vi "Synchronous Trigger (5772).vi"() -> (1 "Trigger":bool[](array[boolean]), 2 "Trigger":u8, 3 "Trig":bool)   [LabVIEW 2012]
uses:
  <vilib>/rvi/eio/common/nirviEmuTemplateMethod_errors.vi
  <vilib>/eio/EIONode/EIONode.xnode
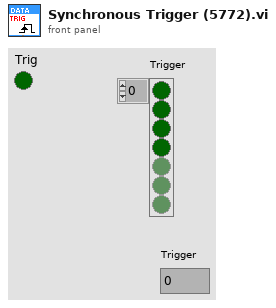
[diagram p1: front panel]
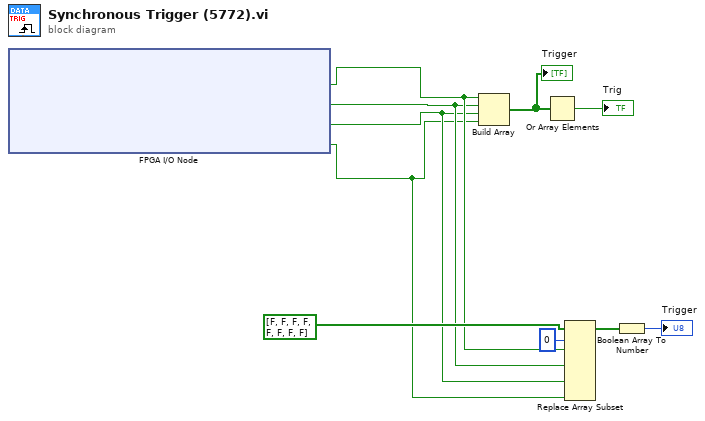
[diagram p0: block diagram]
diagram:
  n1 = xnode "FPGA I/O Node"() -> ("IO Module\\Synchronous Trigger Input N-3"=w7:bool, "IO Module\\Synchronous Trigger Input N-2"=w6:bool, "IO Module\\Synchronous Trigger Input N-1"=w5:bool, "IO Module\\Synchronous Trigger Input N"=w4:bool)  [unwired: 4 in, 4 out]
  n2 = Build Array(w7, w6, w5, w4) -> (w9:bool[])
  "Trigger" <- w9
  n3 = Or Array Elements(Boolean array=w9) -> (logical OR=→"Trig":bool)
  n4 = Replace Array Subset(array=bool[] [FALSE, FALSE, FALSE, FALSE, FALSE, FALSE, FALSE, FALSE], new element #1=w7, index #1=0 ("index"), new element #2=w6, new element #3=w5, new element #4=w4) -> (w2:bool[])  [unwired: 3 in]
  n5 = Boolean Array To Number(Boolean array=w2) -> (number=→"Trigger":u8)
